vi "Handle Value Change.vi"(5 "VolatusAPI":refnum<class "VolatusAPI.lvclass">, 7 "CtlRef":refnum<vi>, 8 "error in (no error)":errorcluster, 9 "NewVal":variant, 10 "OldVal":variant, 11 "LoggingControl in":refnum<class "GroupLoggingControl.lvclass">) -> (0 "error out":errorcluster, 3 "LoggingControl out":refnum<class "GroupLoggingControl.lvclass">)   [LabVIEW 2020, in "VolatusGUIElements.lvlib" / "GroupLoggingControl.lvclass"]
uses:
  GroupLoggingControl.lvclass
  Volatus/VolatusAPI/VolatusAPI.lvclass
  GroupLoggingControl.lvclass/GroupLoggingControl.ctl
  messages/StopLog/Data.ctl
  messages/StopLog/Class/Msg.lvclass/Msg.ctl
  Volatus/VolatusAPI/VolatusAPI.lvclass/VolatusAPI.ctl
  messages/StopLog/Class/Msg.lvclass
  C:/dev/lv20CE/relink/lv-protoc/LV-Proto/Message/Message.lvclass
  lv-vecto/Vecto/TCPMessageService/Send Message.vi
  <vilib>/Utility/error.llb/Error Cluster From Error Code.vi
  Log Prompt Async.vi
  lv-protoc/LV-Proto/Message/Message.lvclass
  messages/StopLog/StopLog.lvlib
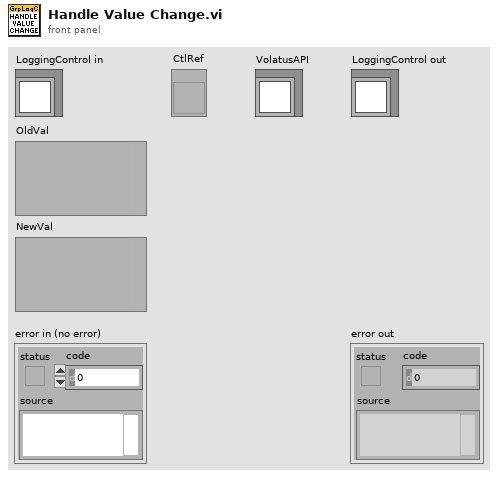
[diagram p1: front panel]
types:
  T1 = typedef "StopLog.lvlib/Data.ctl" = cluster{"reason":string, "groups":string[]}
  T2 = cluster{"Node":string, "Node Color":u32, "Groups":cluster{"Group":string, "Group Color":u32, "Button":bool}[]}[]
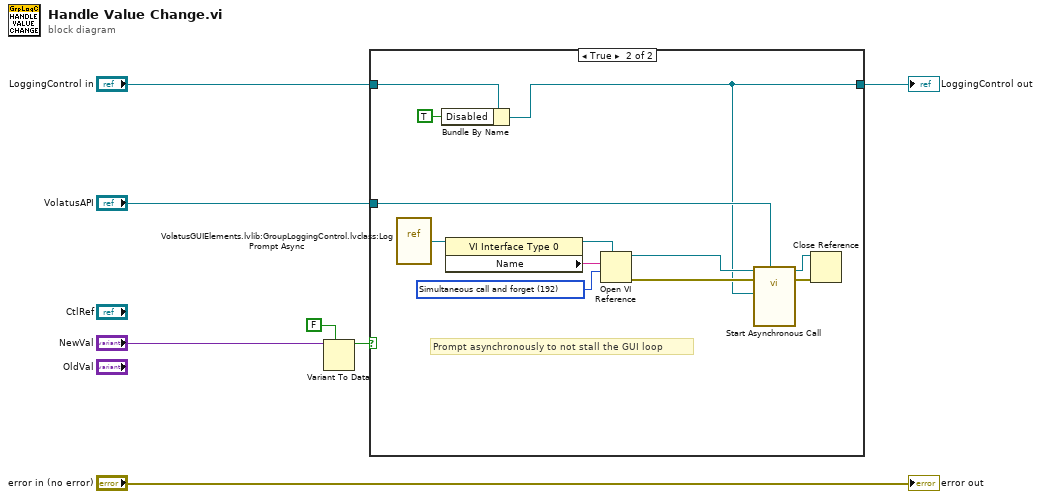
[diagram p0: block diagram]
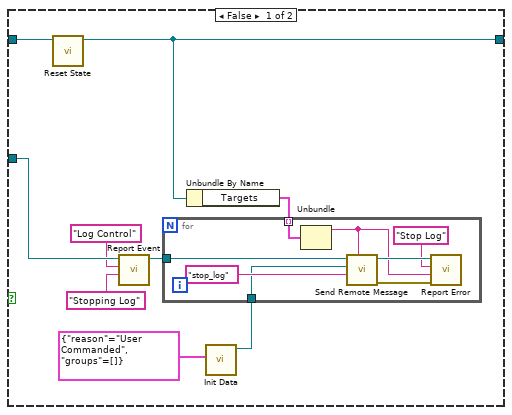
[diagram p2: hidden frame]
diagram:
  n1 = Variant To Data(type=FALSE, Variant="NewVal") -> (data=w1:bool)  [unwired: 1 in, 1 out]
  n2 = case shown="True" w1 {
    tunnel: "VolatusAPI" -> [w16 w28]
    tunnel: "LoggingControl in" -> [w12 w27]
    tunnel: [w11 w26] -> w3
    frame False {
      n3 = call "Reset State.vi"("LoggingControl in"=w12) -> ("LoggingControl out"=w11:refnum<class "GroupLoggingControl.lvclass">)  [unwired: 9 in, 1 out]
      n4 = call "Report Event.vi"("Message"="Stopping Log" ("Context"), "Context"="Log Control", "VolatusAPI in"=w16) -> ("VolatusAPI out"=w10:refnum<class "VolatusAPI.lvclass">)  [unwired: 7 in, 1 out]
      n5 = Unbundle By Name(w11) -> ("Targets"=w13:T2)
      n6 = call "Init Data.vi"("Data"=T1 {"reason"="User Commanded", "groups"=[]}) -> ("Msg out"=w14:refnum<class "Msg.lvclass">)  [unwired: 10 in]
      n7 = for {
        tunnel: w10 -> [w24]
        tunnel: w13 -> [w19] mode=indexing
        tunnel: w14 -> [w18]
        n8 = Unbundle(w19) -> ("Node"=w17:string)  [unwired: 2 out]
        n9 = call "Send Remote Message.vi"("Target Name"=w17, "Message Type"="stop_log", "Message"=w18, "VolatusAPI in"=w24) -> ("error out"=w20:errorcluster, "VolatusAPI out"=w23:refnum<class "VolatusAPI.lvclass">)  [unwired: 6 in]
        n10 = call "Report Error.vi"("error in (no error)"=w20, "Message"=w17, "Context"="Stop Log", "VolatusAPI in"=w23) -> ()  [unwired: 6 in, 2 out]
      }
    }
    frame True {
      w31 = 192 items=["Record modifications"=1, "Open templates for editing"=2, "Prompt user to save"=4, "Prepare for reentrant run"=8, "Prompt to find missing subVIs"=16, "Hide loading dialog box"=32, "Enable simultaneous calls"=64, "Prepare to call and forget"=128, "Simultaneous call and forget"=192, "Prepare to call and collect"=256, "Simultaneous call and collect"=320]
      # "Prompt asynchronously to not stall the GUI loop"
      n11 = vi-ref "VolatusGUIElements.lvlib:GroupLoggingControl.lvclass:Log Prompt Async.vi"() -> (w29:refnum<vi>)
      n12 = Bundle By Name(cluster=w27, "Disabled"=TRUE) -> (w26:refnum<class "GroupLoggingControl.lvclass">)
      n13 = property class="VI Interface Type 0"(reference=w29) -> (reference out=w32:refnum<vi>, "Name"=w30:string)  [unwired: 1 in, 1 out]
      n14 = Open VI Reference(type specifier VI Refnum (for type only)=w32, vi path=w30, options=w31) -> (vi reference=w34:refnum<vi>, error out=w33:errorcluster)  [unwired: 3 in]
      n15 = call-by-ref "Start Asynchronous Call"(reference=w34, error in=w33, "VolatusAPI"=w28, "LoggingControl in"=w26) -> (reference out=w36:refnum<vi>, error out=w35:errorcluster)  [unwired: 10 in]
      n16 = Close Reference(reference=w36, error in (no error)=w35) -> ()  [unwired: 1 out]
    }
  }
  "LoggingControl out" <- w3
  "error out" <- "error in (no error)"
